vi "ReadPointFromMem.vi"(11 "PointNum":u32) -> (3 "Point":cluster{"X":i32, "Y":i32, "Z":i32})   [LabVIEW 2011]
uses:
  <vilib>/Platform/TimedLoop/XDataNode/timing_clust.ctl
  <vilib>/Platform/TimedLoop/XDataNode/nitl_modes.ctl
  <vilib>/Platform/TimedLoop/XDataNode/wakeup.ctl
  <vilib>/rvi/eio/common/nirviEmuTemplateMethod_errors.vi
  <vilib>/Platform/TimedLoop/XDataNode/XDataNode.xnode
  <vilib>/eio/EIONode/EIONode.xnode
  <vilib>/Platform/TimedLoop/XDataNode/XDNodeRunTimeDep.lvlib
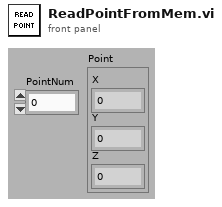
[diagram p1: front panel]
types:
  T1 = typedef "XDNodeRunTimeDep.lvlib/timing_clust.ctl" = cluster{"Expected End [f-1]":u64, "Actual End [f-1]":u64, "Finished Late? [f-1]":bool, "Expected End [i-1]":u64, "Actual End [i-1]":u64, "Finished Late? [i-1]":bool, "Expected Start [i]":u64, "Actual Start [i]":u64, "Expected Start [f]":u64, "Actual Start [f]":u64, "Source Name":string, "Structure Name":string, "Period":i64, "Deadline":i64, "Offset":i64, "Start":i64, "Priority":i32, "Timeout":i32, "Mode":T2, "Wakeup Reason":T3, "Error":errorcluster, "Source Type":string, "Secondary Source Type":string, "Global End Time":u64, "Global Start Time":u64, "Frame Duration":u64, "Iteration Duration":u64, "Assigned CPU":i32, "I/O Scan Engine Mode":u32}
  T2 = typedef "XDNodeRunTimeDep.lvlib/nitl_modes.ctl" = enum32{"No Change", "Process missed periods, maintain original phase", "Discard missed periods, maintain original phase", "Process missed periods, ignore original phase", "Discard missed periods, ignore original phase"}
  T3 = typedef "XDNodeRunTimeDep.lvlib/wakeup.ctl" = enum32{"Normal", "Aborted", "Asynchronous wakeup", "Timing source error", "Timed loop error", "Timeout"}
  T4 = enum16{"ReadXY", "XYstrobe", "ReadZ", "ZStrobe", "Done"}
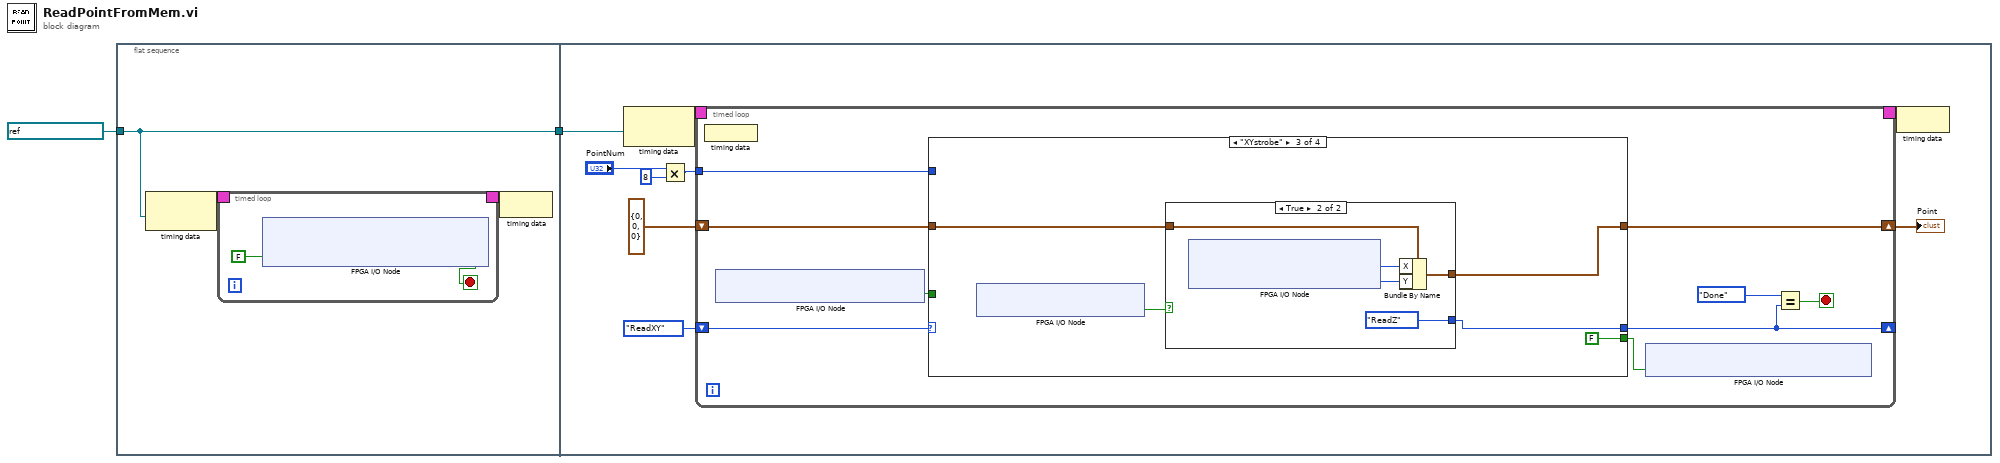
[diagram p0: block diagram]
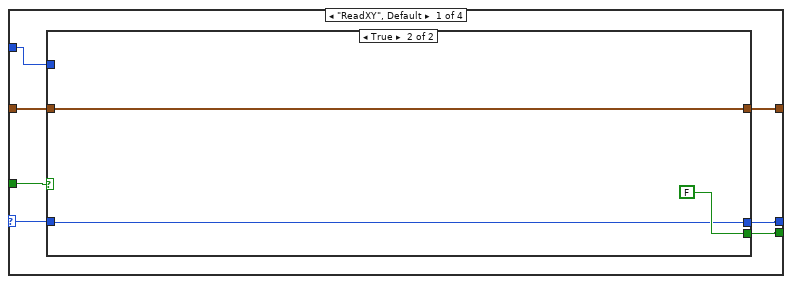
[diagram p2: hidden frame]
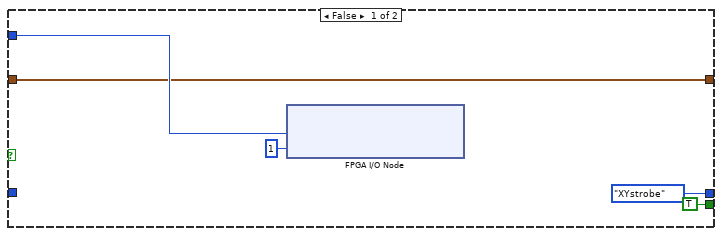
[diagram p3: hidden frame]
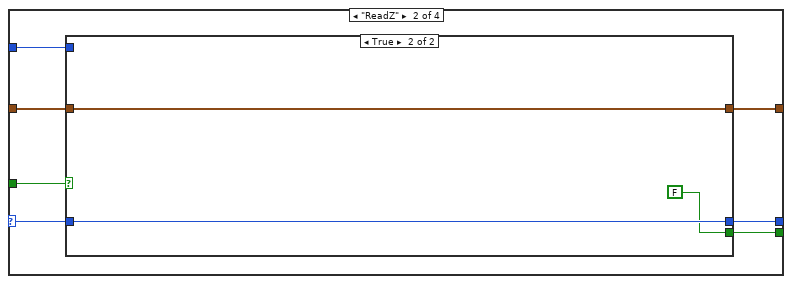
[diagram p4: hidden frame]
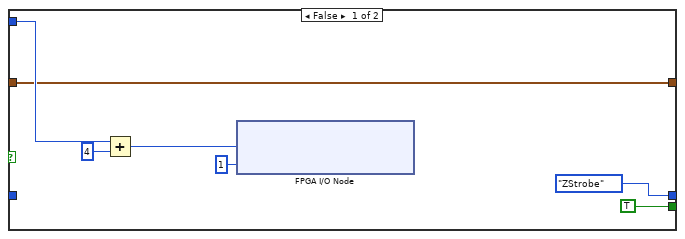
[diagram p5: hidden frame]
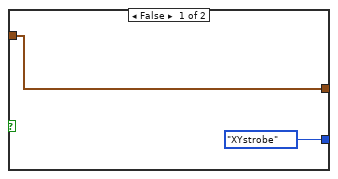
[diagram p6: hidden frame]
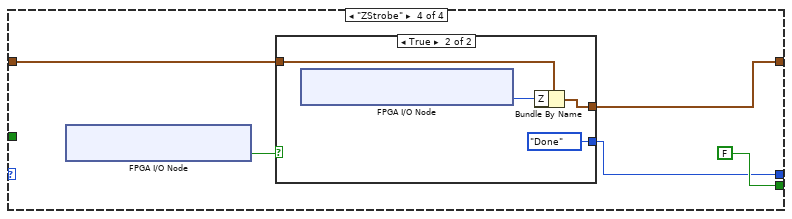
[diagram p7: hidden frame]
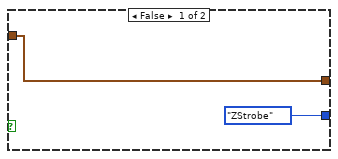
[diagram p8: hidden frame]
diagram:
  n1 = flat-sequence {
    tunnel: refnum<k21> "100 MHz Clock" ("Source Name") -> [w3]
    tunnel: [w3] -> w1
    tunnel: w1 -> [w12]
    frame #0 {
      n2 = node-c288(w3) -> (w5:T1)
      n3 = timed-loop {
        timing: w5 -> [_]
        timing-out: [_] -> w4
        stop <- w7 stop-if-true
        n4 = xnode "FPGA I/O Node"("DRAM Bank 0\\Command_Write_Enable"=FALSE ("DRAM Bank 0\\Command_Write_Enable")) -> ("DRAM Bank 0\\Initialization_Done"=w7:bool)  [unwired: 2 in, 2 out]
      }
      n5 = node-c288(w4) -> ()
    }
    frame #1 {
      n6 = node-c288(w12) -> (w20:T1)
      n7 = Multiply(x="PointNum", y=i16 8) -> (x*y=w16:u32)
      n8 = timed-loop {
        timing: w20 -> [_]
        timing-out: [_] -> w19
        tunnel: w16 -> [w27]
        shift-right: [w23] -> _
        shift-left: T4."ReadXY" -> [w28]
        shift-right: [w25] -> w13
        shift-left: cluster{"X":i32, "Y":i32, "Z":i32} {"X"=0, "Y"=0, "Z"=0} ("Point") -> [w26]
        stop <- w24 stop-if-true
        n9 = node-c288() -> ()  [unwired: 1 in]
        n10 = xnode "FPGA I/O Node"() -> ("DRAM Bank 0\\Command_FIFO_Full"=w21:bool)  [unwired: 1 in, 1 out]
        n11 = case shown="\"XYstrobe\"" w28 {
          selector: w28 -> [w32 w45 _ _]
          tunnel: [w35 w49 w62 w74] -> w23
          tunnel: [w34 w50 FALSE FALSE] -> w29
          tunnel: w27 -> [w36 w51 _ _]
          tunnel: w26 -> [w31 w47 w64 w77]
          tunnel: [w30 w46 w63 w75] -> w25
          tunnel: w21 -> [w33 w48 _ _]
          frame "ReadXY", Default {
            n12 = case shown="True" w33 {
              tunnel: w36 -> [w41 _]
              tunnel: [enum16{"ReadXY", "XYstrobe", "ReadZ", "ZStrobe"}."XYstrobe" w43] -> w35
              tunnel: [TRUE FALSE] -> w34
              tunnel: w32 -> [_ w43]
              tunnel: w31 -> [w37 w42]
              tunnel: [w37 w42] -> w30
              frame False {
                n13 = xnode "FPGA I/O Node"("DRAM Bank 0\\Address"=w41, "DRAM Bank 0\\Command"=u8 1 ("DRAM Bank 0\\Command")) -> ()  [unwired: 2 in, 2 out]
              }
              frame True {
              }
            }
          }
          frame "ReadZ" {
            n14 = case shown="True" w48 {
              tunnel: w51 -> [w57 _]
              tunnel: [TRUE FALSE] -> w50
              tunnel: [enum16{"ReadXY", "XYstrobe", "ReadZ", "ZStrobe"}."ZStrobe" w60] -> w49
              tunnel: w47 -> [w52 w61]
              tunnel: [w52 w61] -> w46
              tunnel: w45 -> [_ w60]
              frame False {
                n15 = Add(x=w57, y=u32 4) -> (x+y=w55:u32)
                n16 = xnode "FPGA I/O Node"("DRAM Bank 0\\Address"=w55, "DRAM Bank 0\\Command"=u8 1 ("DRAM Bank 0\\Command")) -> ()  [unwired: 2 in, 2 out]
              }
              frame True {
              }
            }
          }
          frame "XYstrobe" {
            n17 = xnode "FPGA I/O Node"() -> ("DRAM Bank 0\\Read_Strobe"=w65:bool)  [unwired: 1 in, 1 out]
            n18 = case shown="True" w65 {
              tunnel: w64 -> [w68 w73]
              tunnel: [w68 w70] -> w63
              tunnel: [enum16{"ReadXY", "XYstrobe", "ReadZ", "ZStrobe"}."XYstrobe" enum16{"ReadXY", "XYstrobe", "ReadZ", "ZStrobe"}."ReadZ"] -> w62
              frame False {
              }
              frame True {
                n19 = xnode "FPGA I/O Node"() -> ("DRAM Bank 0\\Read_Data_Upper"=w72:u64, "DRAM Bank 0\\Read_Data_Lower"=w71:u64)  [unwired: 2 in, 2 out]
                n20 = Bundle By Name(cluster=w73, "X"=w72, "Y"=w71) -> (w70:cluster{"X":i32, "Y":i32, "Z":i32})
              }
            }
          }
          frame "ZStrobe" {
            n21 = xnode "FPGA I/O Node"() -> ("DRAM Bank 0\\Read_Strobe"=w78:bool)  [unwired: 1 in, 1 out]
            n22 = case shown="True" w78 {
              tunnel: w77 -> [w80 w84]
              tunnel: [w80 w82] -> w75
              tunnel: [enum16{"ReadXY", "XYstrobe", "ReadZ", "ZStrobe"}."ZStrobe" T4."Done"] -> w74
              frame False {
              }
              frame True {
                n23 = xnode "FPGA I/O Node"() -> ("DRAM Bank 0\\Read_Data_Upper"=w83:u64)  [unwired: 1 in, 1 out]
                n24 = Bundle By Name(cluster=w84, "Z"=w83) -> (w82:cluster{"X":i32, "Y":i32, "Z":i32})
              }
            }
          }
        }
        n25 = xnode "FPGA I/O Node"("DRAM Bank 0\\Command_Write_Enable"=w29) -> ()  [unwired: 1 in, 1 out]
        n26 = Equal?(x=T4."Done", y=w23) -> (x = y?=w24:bool)
      }
      "Point" <- w13
      n27 = node-c288(w19) -> ()
    }
  }
